vi "VNA_Trigger.vi"(2 "error in (no error)":errorcluster, 3 "VISA in":refnum<visa-resource-name>) -> (0 "error out":errorcluster, 1 "VISA out":refnum<visa-resource-name>)   [LabVIEW 2017]
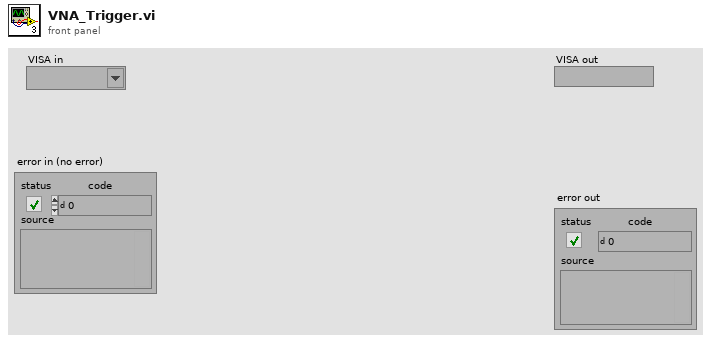
[diagram p1: front panel]
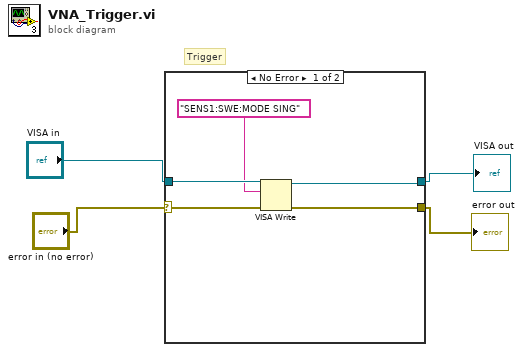
[diagram p0: block diagram]
diagram:
  # "Trigger"
  n1 = case shown="No Error" "error in (no error)" {
    selector: "error in (no error)" -> [w8 w11]
    tunnel: [w5 w11] -> w2
    tunnel: "VISA in" -> [w9 w10]
    tunnel: [w6 w10] -> w4
    frame No Error {
      n2 = VISA Write(VISA resource name=w9, write buffer="SENS1:SWE:MODE SING" ("Cmdline"), error in (no error)=w8) -> (VISA resource name out=w6:refnum<visa-resource-name>, error out=w5:errorcluster)  [unwired: 1 out]
    }
    frame Error {
    }
  }
  "VISA out" <- w4
  "error out" <- w2
